vi "0x2 RIO-OCU command receive.vi"(11 "Manual Override Reader In":refnum<class "NetworkStreamReader.lvclass">) -> (3 "Manual Override Reader Out":refnum<class "NetworkStreamReader.lvclass">)   [LabVIEW 2011]
doc: "Gets commands from the OCU and sends them out to the rest of the code on the RIO using the globals."
uses:
  0x2 Classes/NetworkStreams/Reader/NetworkStreamReader.lvclass
  0x2 Typedefs/ocuCommands.ctl
  0x2 Typedefs/manual override.ctl
  2-Think/2 Typedefs/setpoints to boat.ctl
  2-Think/2 Typedefs/sail setpt.ctl
  2-Think/2 Typedefs/rudder angle.ctl
  0x2 Typedefs/ocuMessage.ctl
  2-Think/2 Classes/Waypoint/Waypoint.lvclass
  2-Think/2 Typedefs/UTM Circle.ctl
  2-Think/2 Classes/Missions/GenericMission/GenericMission.lvclass
  0x2 Typedefs/Current Waypoint.ctl
  0x2 Typedefs/Control values.ctl
  2-Think/2 Typedefs/Goodness Weightings.ctl
  2-Think/2 Typedefs/PI Constants.ctl
  2-Think/2 Typedefs/Apparent Wind Mode.ctl
  0x2 Typedefs/Sail Setting Tuning.ctl
  2-Think/2 Globals/2 Global.vi
  2-Think/2 Globals/2 TuningConstants.vi
  2-Think/2 Globals/2 Message Logger.vi
  2-Think/2 Classes/MissionQueue/MissionQueue.lvclass
  2-Think/2 Classes/Logger/Logger.lvclass
panel:
  out "Latest OCU Command":T1
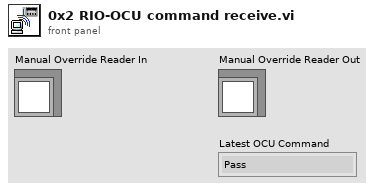
[diagram p1: front panel]
types:
  T1 = typedef "ocuCommands.ctl" = enum16{"Pass", "Send override", "Add waypoint", "Set waypoint number", "Stop", "Add Mission", "Reset Missions/Waypts", "Edit Control Values", "Add Global No-Sail", "Log Message"}
  T2 = typedef "manual override.ctl" = cluster{"Override Active Rudder":bool, "Setpoints":T3, "Override Active Sail":bool}
  T3 = typedef "setpoints to boat.ctl" = cluster{"Sail Position":T4, "Rudder Angle":T5}
  T4 = typedef "sail setpt.ctl" = dbl
  T5 = typedef "rudder angle.ctl" = dbl
  T6 = typedef "ocuMessage.ctl" = cluster{"OCU Command":T1, "Data":variant}
  T7 = typedef "UTM Circle.ctl" = cluster{"UTM Zone":dbl, "Hemisphere":enum16{"North", "South"}, "East":dbl, "North":dbl, "Radius":dbl}
  T8 = typedef "Current Waypoint.ctl" = i32
  T9 = typedef "Control values.ctl" = cluster{"Goodness Weightings":T10, "PI Constants":T11, "No Sail Zone\nTuning Quotient":dbl, "Heading Change Wind Adjustment":dbl, "Waypoint Tuning Quotient":dbl, "Apparent Wind Mode":T12, "RP Autonomous":bool, "Let Sail Out on Windcross":bool, "Shift Goal for currents":bool, "Round Buoy Safety":dbl, "Sail Setting Options":T13, "Defilter Wind Data":bool, "Irons Range":dbl, "Convincing Range":dbl, "Run Range":dbl, "Force tack attempt?":bool, "Minimum\ntack try\ntime?":dbl}
  T10 = typedef "Goodness Weightings.ctl" = cluster{"Target Importance":dbl, "No Sail Importance":dbl, "Change Importance":dbl, "Pure Waypoint \nImportance":dbl, "Pure Wind \nImportance":dbl}
  T11 = typedef "PI Constants.ctl" = cluster{"Proportional Gain":dbl, "Integral Time":dbl, "Derivative Time":dbl}
  T12 = typedef "Apparent Wind Mode.ctl" = cluster{"Desired Apparent\nWind Direction":dbl, "On":bool}
  T13 = typedef "Sail Setting Tuning.ctl" = cluster{"Linear\nMode":bool, "Sails Full In Point":dbl, "Sails Full Out Point":dbl}
  T14 = typedef "Waypoints List.ctl" = refnum<class "Waypoint.lvclass">[]
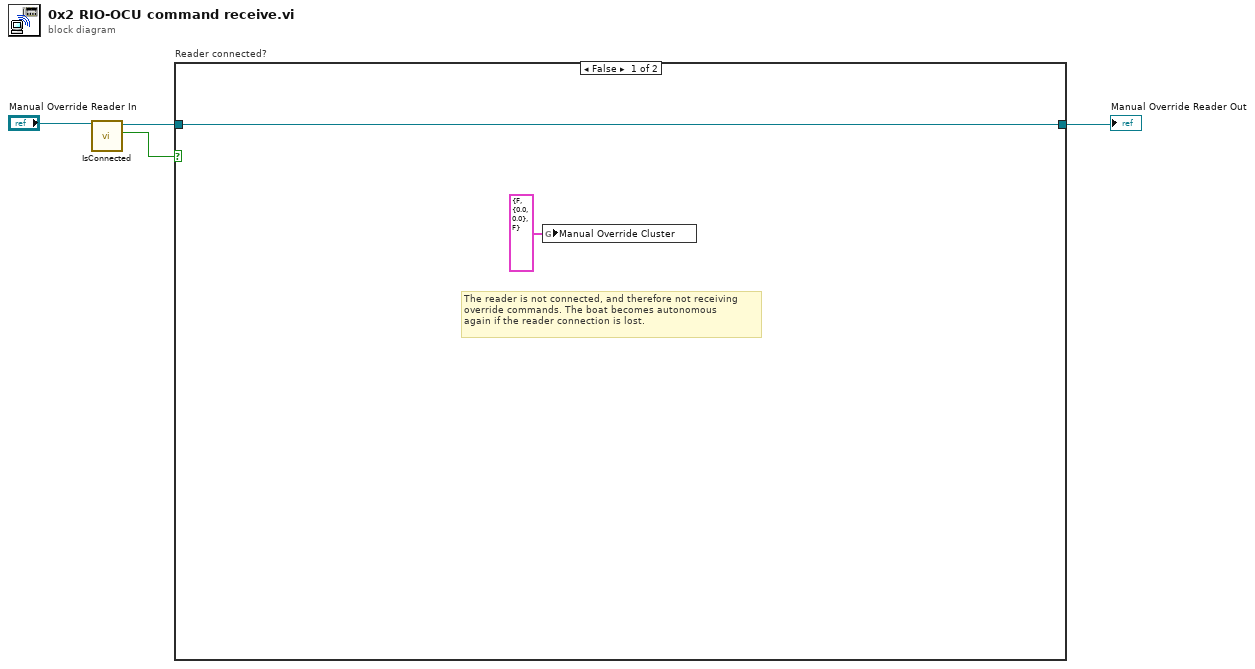
[diagram p0: block diagram]
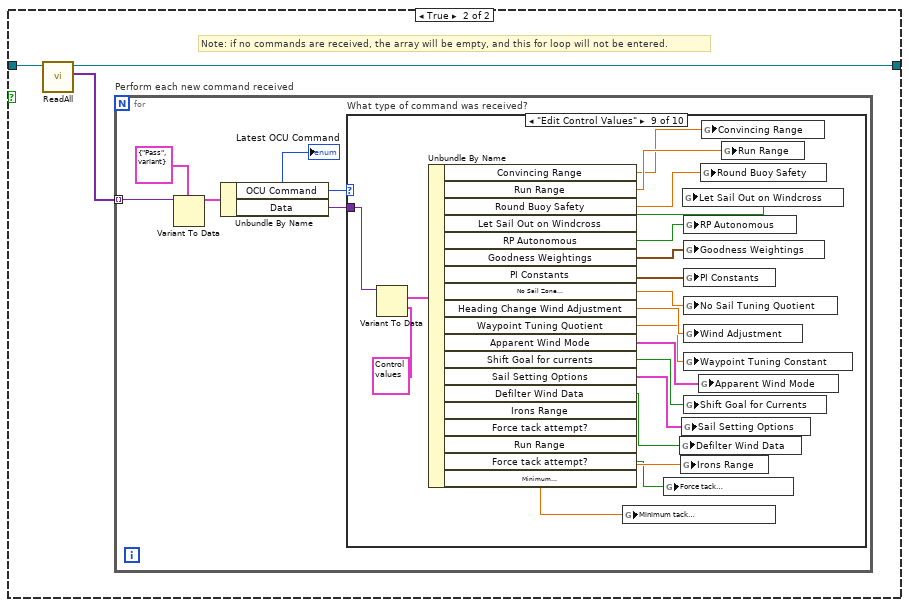
[diagram p2: hidden frame]
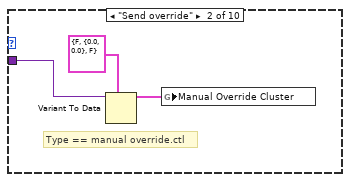
[diagram p4: hidden frame]
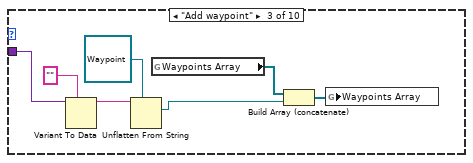
[diagram p5: hidden frame]
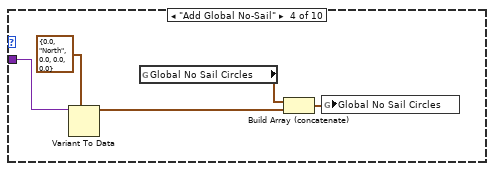
[diagram p6: hidden frame]
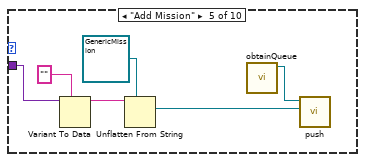
[diagram p7: hidden frame]
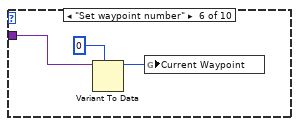
[diagram p8: hidden frame]
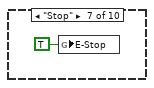
[diagram p9: hidden frame]
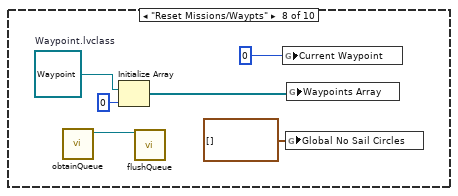
[diagram p10: hidden frame]
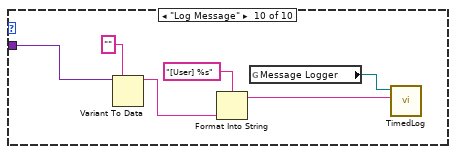
[diagram p11: hidden frame]
diagram:
  n1 = call "IsConnected.vi"("NetworkStreamReader in"="Manual Override Reader In") -> ("Connected?"=w3:bool, "NetworkStreamReader out"=w2:refnum<class "NetworkStreamReader.lvclass">)  [unwired: 8 in, 1 out]
  n2 = case "Reader connected?" shown="False" w3 {
    tunnel: w2 -> [w5 w8]
    tunnel: [w5 w7] -> w1
    frame False {
      # "The reader is not connected, and therefore not receiving\noverride commands. The boat becomes autonomous \nagain if the reader connection is lost."
      n3 = global write "2 Global.vi" "Manual Override Cluster"(T2 {"Override Active Rudder"=FALSE, "Setpoints"={"Sail Position"=0.0, "Rudder Angle"=0.0}, "Override Active Sail"=FALSE} ("Manual Override Cluster")) -> ()
    }
    frame True {
      # "Note: if no commands are received, the array will be empty, and this for loop will not be entered."
      n4 = call "ReadAll.vi"("NetworkStreamReader in"=w8) -> ("elements"=w9:variant[], "NetworkStreamReader out"=w7:refnum<class "NetworkStreamReader.lvclass">)  [unwired: 6 in, 3 out]
      n5 = for "Perform each new command received" {
        tunnel: w9 -> [w10] mode=indexing
        n6 = Variant To Data(type=T6 {"OCU Command"=enum."Pass", "Data"=variant} ("OCU Message"), Variant=w10) -> (data=w13:T6)  [unwired: 1 in, 1 out]
        n7 = Unbundle By Name(w13) -> ("OCU Command"=w12:T1, "Data"=w11:variant)
        "Latest OCU Command" <- w12
        n8 = case "What type of command was received?" shown="\"Edit Control Values\"" w12 {
          tunnel: w11 -> [_ w16 w24 w29 w33 w38 _ _ w65 w70]
          frame "Pass", Default {
          }
          frame "Send override" {
            # "Type == manual override.ctl"
            n9 = Variant To Data(type=T2 {"Override Active Rudder"=FALSE, "Setpoints"={"Sail Position"=0.0, "Rudder Angle"=0.0}, "Override Active Sail"=FALSE} ("Manual Override Cluster"), Variant=w16) -> (data=w15:T2)  [unwired: 1 in, 1 out]
            n10 = global write "2 Global.vi" "Manual Override Cluster"(w15) -> ()
          }
          frame "Add waypoint" {
            n11 = Variant To Data(type="", Variant=w24) -> (data=w20:string)  [unwired: 1 in, 1 out]
            n12 = Unflatten From String(type=refnum<class "Waypoint.lvclass"> refnum ("Waypoint.lvclass"), binary string=w20) -> (value=w18:refnum<class "Waypoint.lvclass">)  [unwired: 3 in, 2 out]
            n13 = global read "2 Global.vi" "Waypoints Array"() -> (w23:T14)
            n14 = Build Array (concatenate)(w23, w18) -> (w22:T14)
            n15 = global write "2 Global.vi" "Waypoints Array"(w22) -> ()
          }
          frame "Add Global No-Sail" {
            n16 = Variant To Data(type=T7 {"UTM Zone"=0.0, "Hemisphere"=enum."North", "East"=0.0, "North"=0.0, "Radius"=0.0} ("UTM Location"), Variant=w29) -> (data=w25:T7)  [unwired: 1 in, 1 out]
            n17 = global read "2 Global.vi" "Global No Sail Circles"() -> (w28:T7[])
            n18 = Build Array (concatenate)(w28, w25) -> (w27:T7[])
            n19 = global write "2 Global.vi" "Global No Sail Circles"(w27) -> ()
          }
          frame "Add Mission" {
            n20 = Variant To Data(type="", Variant=w33) -> (data=w34:string)  [unwired: 1 in, 1 out]
            n21 = Unflatten From String(type=refnum<class "GenericMission.lvclass"> refnum ("GenericMission.lvclass"), binary string=w34) -> (value=w30:refnum<class "GenericMission.lvclass">)  [unwired: 3 in, 2 out]
            n22 = call "obtainQueue.vi"() -> ("MissionQueue.lvclass"=w31:refnum<class "MissionQueue.lvclass">)  [unwired: 10 in, 1 out]
            n23 = call "push.vi"("GenericMission.lvclass"=w30, "MissionQueue in"=w31) -> ()  [unwired: 8 in, 2 out]
          }
          frame "Set waypoint number" {
            n24 = Variant To Data(type=T8 0 ("Current Waypoint"), Variant=w38) -> (data=w36:T8)  [unwired: 1 in, 1 out]
            n25 = global write "2 Global.vi" "Current Waypoint"(w36) -> ()
          }
          frame "Stop" {
            n26 = global write "2 Global.vi" "E-Stop"(TRUE ("E-Stop")) -> ()
          }
          frame "Reset Missions/Waypts" {
            w42 = refnum<class "Waypoint.lvclass"> refnum  # Waypoint.lvclass
            n27 = call "obtainQueue.vi"() -> ("MissionQueue.lvclass"=w41:refnum<class "MissionQueue.lvclass">)  [unwired: 10 in, 1 out]
            n28 = Initialize Array(w42, 0 ("dimension size")) -> (w44:refnum<class "Waypoint.lvclass">[])
            n29 = call "flushQueue.vi"("MissionQueue in"=w41) -> ()  [unwired: 8 in, 3 out]
            n30 = global write "2 Global.vi" "Current Waypoint"(T8 0 ("Current Waypoint")) -> ()
            n31 = global write "2 Global.vi" "Global No Sail Circles"(T7[] [] ("Global No Sail Circles")) -> ()
            n32 = global write "2 Global.vi" "Waypoints Array"(w44) -> ()
          }
          frame "Edit Control Values" {
            n33 = Variant To Data(type=T9 {"Goodness Weightings"={"Target Importance"=0.0, "No Sail Importance"=0.0, "Change Importance"=0.0, "Pure Waypoint \nImportance"=0.0, "Pure Wind \nImportance"=0.0}, "PI Constants"={"Proportional Gain"=0.0, "Integral Time"=0.0, "Derivative Time"=0.0}, "No Sail Zone\nTuning Quotient"=0.0, "Heading Change Wind Adjustment"=0.0, "Waypoint Tuning Quotient"=0.0, "Apparent Wind Mode"={"Desired Apparent\nWind Direction"=0.0, "On"=FALSE}, "RP Autonomous"=FALSE, "Let Sail Out on Windcross"=FALSE, "Shift Goal for currents"=FALSE, "Round Buoy Safety"=0.0, "Sail Setting Options"={"Linear\nMode"=FALSE, "Sails Full In Point"=0.0, "Sails Full Out Point"=0.0}, "Defilter Wind Data"=FALSE, "Irons Range"=0.0, "Convincing Range"=0.0, "Run Range"=0.0, "Force tack attempt?"=FALSE, "Minimum\ntack try\ntime?"=0.0}, Variant=w65) -> (data=w64:T9)  [unwired: 1 in, 1 out]
            n34 = Unbundle By Name(w64) -> ("Convincing Range"=w48:dbl, "Run Range"=w49:dbl, "Round Buoy Safety"=w53:dbl, "Let Sail Out on Windcross"=w55:bool, "RP Autonomous"=w56:bool, "Goodness Weightings"=w62:T10, "PI Constants"=w61:T11, "No Sail Zone\nTuning Quotient"=w63:dbl, "Heading Change Wind Adjustment"=w60:dbl, "Waypoint Tuning Quotient"=w59:dbl, "Apparent Wind Mode"=w57:T12, "Shift Goal for currents"=w54:bool, "Sail Setting Options"=w52:T13, "Defilter Wind Data"=w51:bool, "Irons Range"=w50:dbl, "Force tack attempt?"=w47:bool, "Minimum\ntack try\ntime?"=w46:dbl)  [unwired: 2 out]
            n35 = global write "2 TuningConstants.vi" "Minimum tack\ntry time?"(w46) -> ()
            n36 = global write "2 TuningConstants.vi" "Force tack\nattempt?"(w47) -> ()
            n37 = global write "2 Global.vi" "Defilter Wind Data"(w51) -> ()
            n38 = global write "2 TuningConstants.vi" "Irons Range"(w50) -> ()
            n39 = global write "2 TuningConstants.vi" "Sail Setting Options"(w52) -> ()
            n40 = global write "2 Global.vi" "Let Sail Out on Windcross"(w55) -> ()
            n41 = global write "2 Global.vi" "RP Autonomous"(w56) -> ()
            n42 = global write "2 TuningConstants.vi" "Goodness Weightings"(w62) -> ()
            n43 = global write "2 TuningConstants.vi" "PI Constants"(w61) -> ()
            n44 = global write "2 TuningConstants.vi" "No Sail Tuning Quotient"(w63) -> ()
            n45 = global write "2 TuningConstants.vi" "Wind Adjustment"(w60) -> ()
            n46 = global write "2 TuningConstants.vi" "Waypoint Tuning Constant"(w59) -> ()
            n47 = global write "2 Global.vi" "Shift Goal for Currents"(w54) -> ()
            n48 = global write "2 TuningConstants.vi" "Apparent Wind Mode"(w57) -> ()
            n49 = global write "2 Global.vi" "Round Buoy Safety"(w53) -> ()
            n50 = global write "2 Global.vi" "Convincing Range"(w48) -> ()
            n51 = global write "2 Global.vi" "Run Range"(w49) -> ()
          }
          frame "Log Message" {
            n52 = Variant To Data(type="" ("Message"), Variant=w70) -> (data=w67:string)  [unwired: 1 in, 1 out]
            n53 = Format Into String(format string="[User] %s", w67) -> (resulting string=w66:string)  [unwired: 2 in, 1 out]
            n54 = global read "2 Message Logger.vi" "Message Logger"() -> (w69:refnum<class "Logger.lvclass">)
            n55 = call "TimedLog.vi"("Message"=w66, "Logger in"=w69) -> ()  [unwired: 7 in, 3 out]
          }
        }
      }
    }
  }
  "Manual Override Reader Out" <- w1
